vi "remove channel from configuration.vi"(5 "channels":refnum<vi>, 7 "user event":T1, 8 "error in":errorcluster, 9 "channels value":i32, 10 "engine configuration in":refnum<class "engine configuration.lvclass">, 11 "Scan Engine configuration in":refnum<class "Scan Engine configuration.lvclass">) -> (0 "error out":errorcluster, 2 "engine configuration out":refnum<class "engine configuration.lvclass">, 3 "Scan Engine configuration out":refnum<class "Scan Engine configuration.lvclass">)   [LabVIEW 2013, in "Scan Engine editor node.lvclass"]
uses:
  Scan Engine editor node.lvclass
  <vilib>/NI/Module Execution Interface/Engine Configuration/engine configuration.lvclass
  module/configuration/Scan Engine configuration.lvclass
  <vilib>/NI/Configuration Framework/Node/UserEventRef.ctl
  <vilib>/NI/Configuration Framework/Controls/EventCluster.ctl
  <vilib>/NI/Configuration Framework/serializable configuration/NISE_CEF_serializable configuration.lvclass/NISE_CEF_serializable configuration.ctl
  <vilib>/Utility/LVClass/Get LV Class Name.vi
  <vilib>/NI/Configuration Framework/error generator/NISE_error generator.vi
  <vilib>/NI/Configuration Framework/NISE_CEF_TreeControl.lvlib
  <vilib>/NI/Configuration Framework/serializable configuration/NISE_CEF_serializable configuration.lvclass
  <vilib>/NI/Configuration Framework/Node/NISE_CEF_Node.lvclass
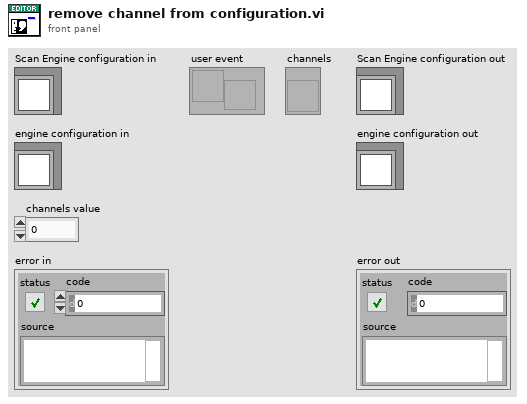
[diagram p1: front panel]
types:
  T1 = typedef "NISE_CEF_Node.lvclass/UserEventRef.ctl" = refnum<user-event>
  T2 = typedef "Scan Engine editor node.lvclass/table line.ctl" = cluster{"tag":string, "channel":refnum<class "TBM channel.lvclass">}
  T3 = typedef "NISE_CEF_TreeControl.lvlib/EventCluster.ctl" = cluster{"command":string, "data":string}
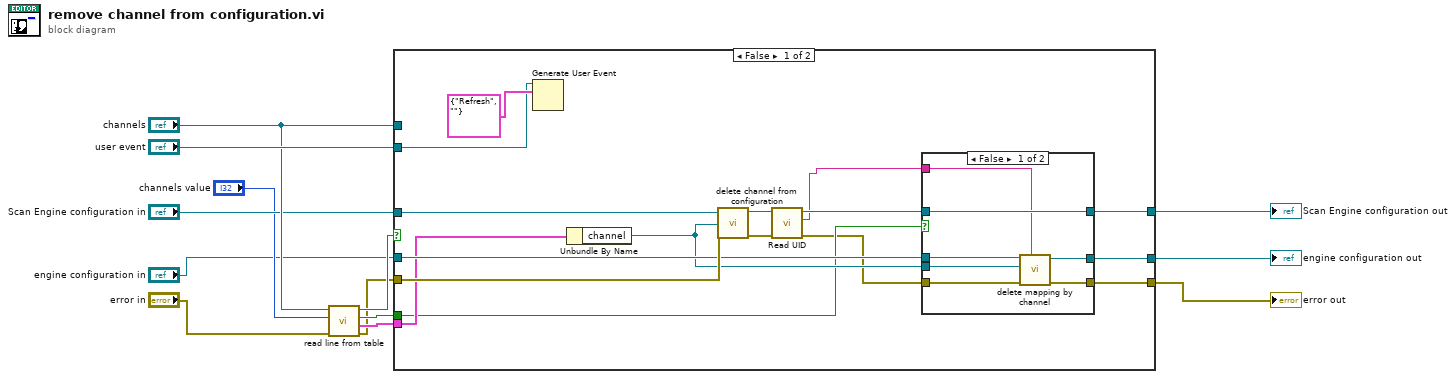
[diagram p0: block diagram]
diagram:
  n1 = call "read line from table.vi"("error in"="error in", "line number"="channels value", "operations table"="channels") -> ("error out"=w4:errorcluster, "line"=w7:T2, "empty tag?"=w9:bool, "empty channel?"=w8:bool)  [unwired: 5 in]
  n2 = case shown="False" w8 {
    tunnel: w4 -> [w28 w40]
    tunnel: "Scan Engine configuration in" -> [w27 w42]
    tunnel: "engine configuration in" -> [w26 w41]
    tunnel: [w25 w41] -> w13
    tunnel: [w21 w42] -> w12
    tunnel: [w24 w40] -> w6
    tunnel: w7 -> [w23 _]
    tunnel: w9 -> [w20 _]
    tunnel: "channels" -> [_ _]
    tunnel: "user event" -> [w18 _]
    frame False {
      n3 = Generate User Event(user event=w18, event data cluster=T3 {"command"="Refresh", "data"=""} ("event data")) -> ()  [unwired: 2 in, 2 out]
      n4 = Unbundle By Name(w23) -> ("channel"=w22:refnum<class "TBM channel.lvclass">)
      n5 = call "delete channel from configuration.vi"("error in"=w28, "channel"=w22, "Scan Engine configuration in"=w27) -> ("error out"=w29:errorcluster, "Scan Engine configuration out"=w16:refnum<class "Scan Engine configuration.lvclass">)  [unwired: 7 in]
      n6 = call <vilib>:"Read UID.vi"("error in"=w29, "configuration in"=w16) -> ("error out"=w17:errorcluster, "instance id"=w14:string, "configuration out"=w15:refnum<class "Scan Engine configuration.lvclass">)  [unwired: 7 in]
      n7 = case shown="False" w20 {
        tunnel: w17 -> [w36 w37]
        tunnel: w26 -> [w35 w39]
        tunnel: [w34 w39] -> w25
        tunnel: [w33 w37] -> w24
        tunnel: w14 -> [w30 _]
        tunnel: w22 -> [w32 _]
        tunnel: [w31 w38] -> w21
        tunnel: w15 -> [w31 w38]
        frame False {
          n8 = call <vilib>:"delete mapping by channel.vi"("owner ID"=w30, "error in"=w36, "channel"=w32, "engine configuration in"=w35) -> ("error out"=w33:errorcluster, "engine configuration out"=w34:refnum<class "engine configuration.lvclass">)  [unwired: 6 in]
        }
        frame True {
        }
      }
    }
    frame True {
    }
  }
  "engine configuration out" <- w13
  "Scan Engine configuration out" <- w12
  "error out" <- w6
